vi "DPDTdll.vi"(8 "error in (no error)":errorcluster, 9 "z":dbl[](array[numeric]), 10 "D":dbl, 11 "t":dbl) -> (0 "error out":errorcluster, 3 "dPdT out":dbl)   [LabVIEW 2016]
doc: "subroutine DPDT (t,D,z,dpt)\n\nCompute partial derivative of pressure w.r.t. temperature at constant\ndensity as a function of temperature, density, and composition\n\nINPUTS:\nt -- temperature [K]\nD -- molar density [mol/L]\nz -- composition [array of mol frac]\n\nOUTPUT:\ndpt -- dP/dT [kPa/K]"
uses:
  REFPROP.DLL
panel:
  # "REFPROP-DPDTdll.vi"
  # "void  DPDTdll(double *t, double *D, double *z, double *dpt)"
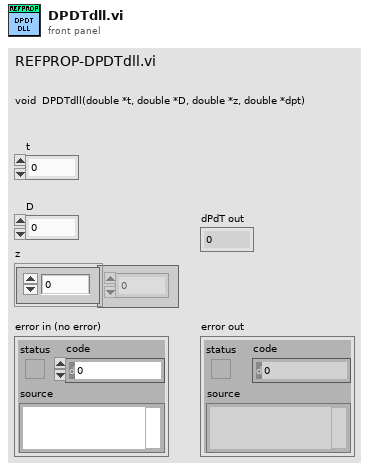
[diagram p1: front panel]
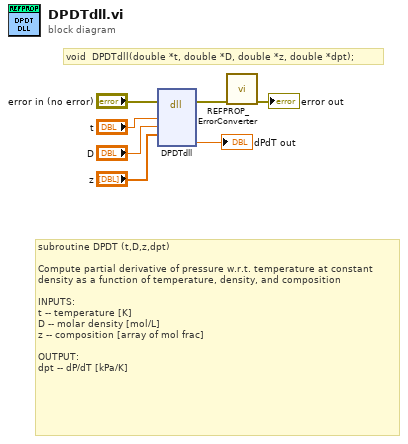
[diagram p0: block diagram]
diagram:
  # "void  DPDTdll(double *t, double *D, double *z, double *dpt);"
  # "subroutine DPDT (t,D,z,dpt)\n\nCompute partial derivative of pressure w.r.t. temperature at constant\ndensity as a function of temperature, density, and composition\n\nINPUTS:\nt -- temperature [K]\nD -- molar density [mol/L]\nz -- composition [array of mol frac]\n\nOUTPUT:\ndpt -- dP/dT [kPa/K]"
  n1 = dll-call lib="S:/009 - Testing/02 - Performance Testing/REFPROP/REFPROP.*" fn="DPDTdll"(error in="error in (no error)", "t"="t", "D"="D", "z"="z") -> (error out=w3:errorcluster, "dpt"=→"dPdT out":dbl)  [unwired: 7 in, 1 out]
  n2 = call "REFPROP_ErrorConverter.vi"("error in (no error)"=w3) -> ("error out"=→"error out":errorcluster)  [unwired: 10 in]
